vi "Create Option with Shared Approval.vi"(10 "Filename":string, 11 "Options In":refnum<class "Options.lvclass">) -> (3 "Options outs":refnum<class "Options.lvclass">)   [LabVIEW 2020]
uses:
  Source/Approval Tests/Options/Options.lvclass
  Source/Approval Tests/Namer With Shared Approved File/Namer With Shared Approved File.lvclass
  C:/Users/SAS/Desktop/ApprovalTests.LabVIEW/Source/Approval Tests/Namer/Namer.lvclass
  Source/Approval Tests/Namer With Shared Approved File/Namer With Shared Approved File.lvclass/Namer With Shared Approved File.ctl
  Source/Approval Tests/Options/Options.lvclass/Options.ctl
  Source/Approval Tests/Namer With Shared Approved File/Write Shared Approved File Path.vi
  Source/Approval Tests/Options/Write Namer.vi
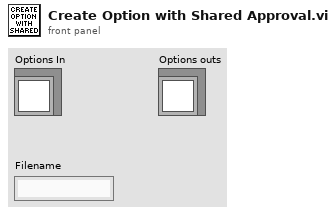
[diagram p1: front panel]
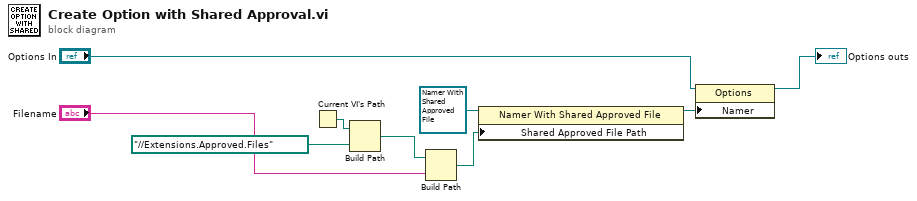
[diagram p0: block diagram]
diagram:
  n1 = Current VI's Path() -> (path=w9:path)
  n2 = Build Path(base path=w9, name or relative path=path "../../Extensions.Approved.Files") -> (appended path=w4:path)
  n3 = Build Path(base path=w4, name or relative path="Filename") -> (appended path=w2:path)
  n4 = property class="Namer With Shared Approved File"(reference=refnum<class "Namer With Shared Approved File.lvclass"> refnum ("Approval Tests.lvlib:Regex Scrubber"), "Shared Approved File Path"=w2) -> (reference out=w7:refnum<class "Namer With Shared Approved File.lvclass">)  [unwired: 1 in, 1 out]
  n5 = property class="Options"(reference="Options In", "Namer"=w7) -> (reference out=→"Options outs":refnum<class "Options.lvclass">)  [unwired: 1 in, 1 out]
